vi "set_params.vi"(8 "error in (no error)":errorcluster caption="entrée d'erreur (pas d'erreur)", 11 "Isomap.lvclass 2":refnum<class "Isomap.lvclass">) -> (0 "error out":errorcluster caption="sortie d'erreur", 3 "Isomap.lvclass":refnum<class "Isomap.lvclass">)   [LabVIEW 2020, in "Isomap.lvclass"]
uses:
  Isomap.lvclass
  Isomap.lvclass/Isomap.ctl
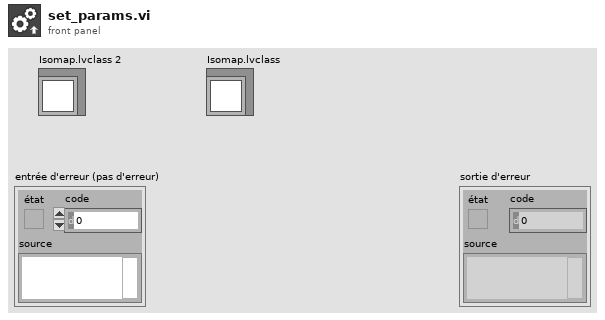
[diagram p1: front panel]
types:
  T1 = typedef "isomap_params.ctl" = cluster{"n_neighbors":dbl, "n_components":dbl, "eigen_solver":string, "tol":dbl, "max_iter":cluster{"max_iter_type":string, "max_iter_int":dbl}, "path_method":string, "neighbors_algorithm":string, "n_jobs":dbl, "metric":cluster{"metric_type":string, "metric_function":string}, "p":dbl}
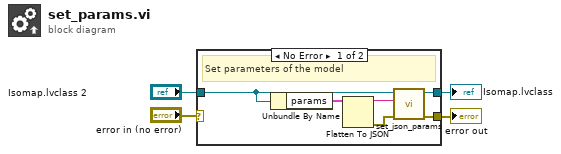
[diagram p0: block diagram]
diagram:
  n1 = case shown="No Error" "error in (no error)" {
    selector: "error in (no error)" -> [_ w12]
    tunnel: [w7 w12] -> w3
    tunnel: [w8 w11] -> w1
    tunnel: "Isomap.lvclass 2" -> [w5 w11]
    frame No Error {
      # "Set parameters of the model"
      n2 = Unbundle By Name(w5) -> ("params"=w10:T1)
      n3 = Flatten To JSON(anything=w10) -> (JSON string=w9:string, 11:w6:errorcluster)  [unwired: 2 in]
      n4 = call-dynamic "set_json_params.vi"("error in (no error)"=w6, "params"=w9, "Model en entrée"=w5) -> ("error out"=w7:errorcluster, "Model en sortie"=w8:refnum<class "Isomap.lvclass">)  [unwired: 7 in]
    }
    frame Error {
    }
  }
  "error out" <- w3
  "Isomap.lvclass" <- w1
